vi "Get Folder.vi"(8 "error in (no error)":errorcluster, 11 "Comp Trace Controller in":refnum<class "Comp Trace Controller.lvclass">) -> (0 "error out":errorcluster, 1 "Folder Found?":bool, 2 "Folder":path, 3 "Comp Trace Controller out":refnum<class "Comp Trace Controller.lvclass">)   [LabVIEW 2014, in "Comp Trace Controller.lvlib" / "Comp Trace Controller.lvclass"]
uses:
  Comp Trace Controller.lvclass
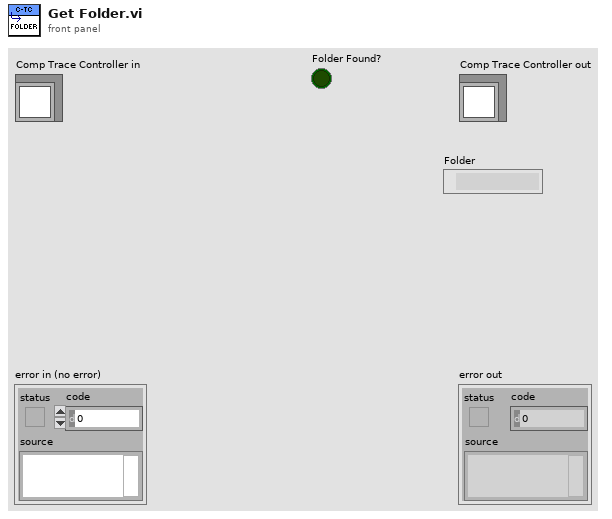
[diagram p1: front panel]
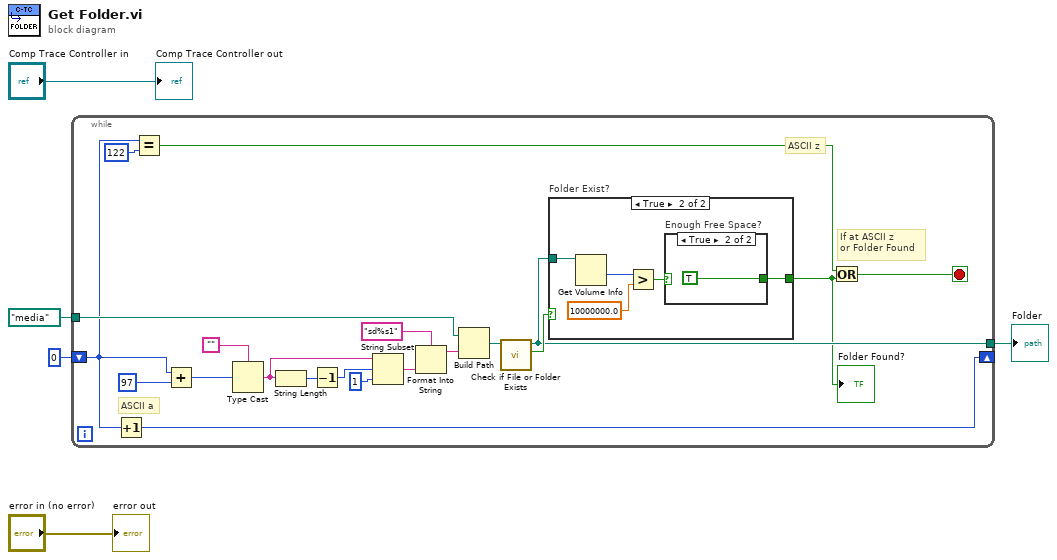
[diagram p0: block diagram]
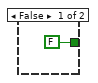
[diagram p2: hidden frame]
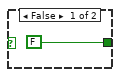
[diagram p3: hidden frame]
diagram:
  n1 = while {
    shift-right: [w20] -> _
    shift-left: 0 -> [w18]
    tunnel: path "/media" ("Folder") -> [w24]
    tunnel: [w7] -> w1
    stop <- w21 stop-if-true
    # "If at ASCII z\nor Folder Found"
    # "ASCII a"
    # "ASCII z"
    n2 = Increment(x=w18) -> (x+1=w20:i32)
    n3 = Equal?(x=w18, y=122) -> (x = y?=w19:bool)
    n4 = Add(x=w18, y=97) -> (x+y=w16:i32)
    n5 = Type Cast(type="", x=w16) -> (*(type *) &x=w12:string)
    n6 = String Length(string=w12) -> (length=w11:i32)
    n7 = Decrement(x=w11) -> (x-1=w10:i32)
    n8 = String Subset(string=w12, offset (0)=w10, length (rest)=1 ("length (rest)")) -> (substring=w13:string)
    n9 = Format Into String(format string="sd%s1", w13) -> (resulting string=w23:string)  [unwired: 2 in, 1 out]
    n10 = Build Path(base path=w24, name or relative path=w23) -> (appended path=w22:path)
    n11 = call <vilib>:"Check if File or Folder Exists.vi"("path"=w22) -> ("file or folder exists?"=w8:bool, "dup path"=w7:path)  [unwired: 8 in, 1 out]
    n12 = case "Folder Exist?" shown="True" w8 {
      tunnel: w7 -> [_ w27]
      tunnel: [FALSE w28] -> w6
      frame False {
      }
      frame True {
        n13 = Get Volume Info(11:w27) -> (1:w31:i64)  [unwired: 1 in, 5 out]
        n14 = Greater?(x=w31, y=10000000.0) -> (0:w30:bool)
        n15 = case "Enough Free Space?" shown="True" w30 {
          tunnel: [FALSE TRUE] -> w28
          frame False {
          }
          frame True {
          }
        }
      }
    }
    "Folder Found?" <- w6
    n16 = Or(x=w19, y=w6) -> (x .or. y?=w21:bool)
  }
  "Folder" <- w1
  "error out" <- "error in (no error)"
  "Comp Trace Controller out" <- "Comp Trace Controller in"
